vi "finishUp.vi"(8 "error in (no error)":errorcluster, 11 "CameraControlViewer in":refnum<class "CameraControlViewer.lvclass">) -> (0 "error out":errorcluster, 3 "CameraControlViewer out":refnum<class "CameraControlViewer.lvclass">)   [LabVIEW 2011, in "Views.lvlib" / "Camera.lvlib" / "CameraControlViewer.lvclass"]
uses:
  CameraControlViewer.lvclass
  CameraControlViewer.lvclass/CameraControlViewer.ctl
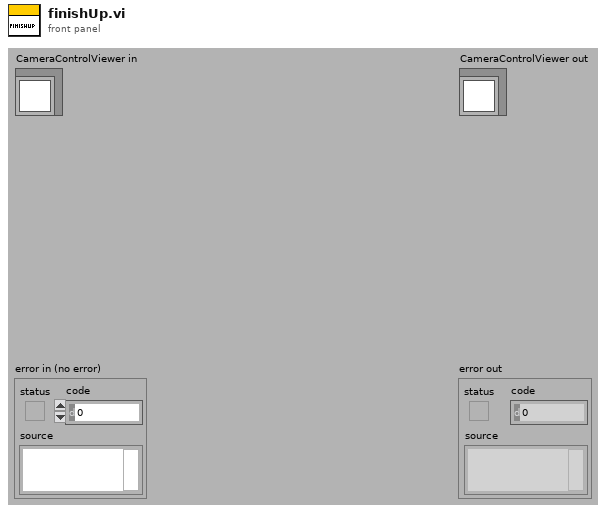
[diagram p1: front panel]
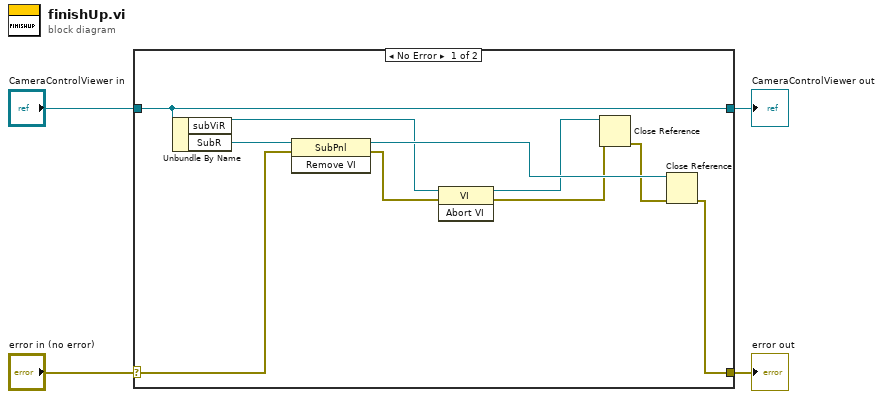
[diagram p0: block diagram]
diagram:
  n1 = case shown="No Error" "error in (no error)" {
    selector: "error in (no error)" -> [w12 w16]
    tunnel: [w9 w16] -> w3
    tunnel: [w14 w15] -> w1
    tunnel: "CameraControlViewer in" -> [w14 w15]
    frame No Error {
      n2 = Unbundle By Name(w14) -> ("subViR"=w8:refnum<vi>, "SubR"=w13:refnum<vi>)
      n3 = invoke class="SubPnl" method="Remove VI"(reference=w13, error in=w12) -> (reference out=w11:refnum<vi>, error out=w7:errorcluster)  [unwired: 1 in, 1 out]
      n4 = invoke class="VI" method="Abort VI"(reference=w8, error in=w7) -> (reference out=w6:refnum<vi>, error out=w5:errorcluster)  [unwired: 1 in, 1 out]
      n5 = Close Reference(reference=w6, error in (no error)=w5) -> (error out=w10:errorcluster)
      n6 = Close Reference(reference=w11, error in (no error)=w10) -> (error out=w9:errorcluster)
    }
    frame Error {
    }
  }
  "error out" <- w3
  "CameraControlViewer out" <- w1
